vi "Set Out.vi"(8 "error in":errorcluster, 11 "6512 in":refnum<class "6512.lvclass">) -> (0 "error out":errorcluster, 3 "6512 out":refnum<class "6512.lvclass">)   [LabVIEW 2019, in "6512.lvlib" / "6512.lvclass"]
uses:
  Library/6512.lvclass
  C:/Users/Public/Documents/Development/builds/Instruments/DIG_IO.lvlibp/Library/DIG_IO.lvclass
  Library/6512.lvclass/6512.ctl
  <vilib>/DAQmx/write.llb/DAQmx Write (Digital 1D U8 NChan 1Samp).vi
  builds/Instruments/DIG_IO.lvlibp/Accessors/Read Digital.vi
  <vilib>/DAQmx/miscellaneous.llb/DAQmx Fill In Error Info.vi
  builds/Engine/Engine.lvlibp/Project/Engine.lvclass
  C:/Users/Public/Documents/Development/builds/Engine/Engine.lvlibp/Project/Engine.lvclass
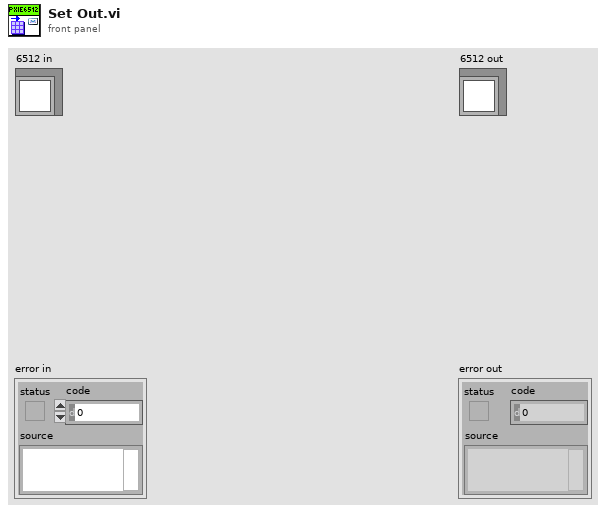
[diagram p1: front panel]
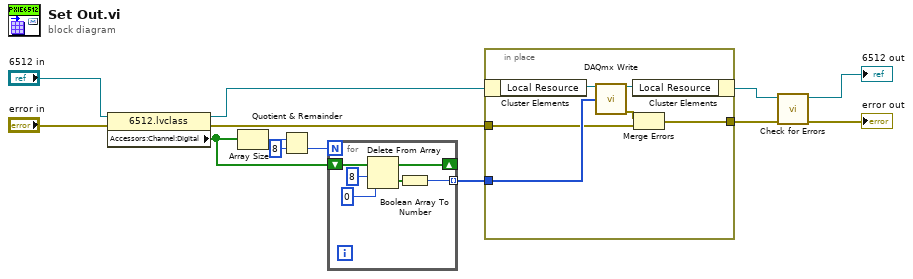
[diagram p0: block diagram]
diagram:
  n1 = property class="6512.lvclass"(reference="6512 in", error in="error in") -> (reference out=w2:refnum<class "6512.lvclass">, error out=w13:errorcluster, "Accessors:Channel:Digital"=w4:bool[])
  n2 = Array Size(array=w4) -> (size(s)=w6:i32)
  n3 = Quotient & Remainder(x=w6, y=8) -> (floor(x/y)=w5:i32)  [unwired: 1 out]
  n4 = for {
    N: w5 -> [_]
    shift-right: [w18] -> _
    shift-left: w4 -> [w19]
    tunnel: [w14] -> w3 mode=indexing
    n5 = Delete From Array(array=w19, length=8, index=0) -> (deleted portion=w15:bool[], array with subset deleted=w18:bool[])
    n6 = Boolean Array To Number(Boolean array=w15) -> (number=w14:u8)
  }
  n7 = in-place {
    in-place-border: w13 -> [w20]
    in-place-border: [w21] -> w10
    in-place-border: w3 -> [w24]
    n8 = in-place-cluster #1(w2) -> ("Local Resource"=w23:refnum<k21>)
    n9 = call-poly <vilib>:"DAQmx Write.vi"("task/channels in"=w23, "data"=w24) -> ("task out"=w22:refnum<k21>, "error out"=w25:errorcluster)  [unwired: 11 in, 1 out]
    n10 = in-place-cluster #1("Local Resource"=w22) -> (w1:refnum<class "6512.lvclass">)
    n11 = Merge Errors(w25, w20) -> (w21:errorcluster)
  }
  n12 = call "Check for Errors.vi"("error in"=w10, "Engine in"=w1) -> ("error out"=→"error out":errorcluster, "Engine out"=→"6512 out":refnum<class "6512.lvclass">)  [unwired: 8 in]
